vi "on_axis_coupling.vi"(11 "Sense coupling":T1 format="%#_3p") -> (3 "Sense amplitudes":T1 format="%#_3p")   [LabVIEW 2026]
uses:
  coupling_matrix.ctl
panel:
  # "Take a current sense coupling matrix and turn it into one suitable for normalization.   The idea is that only the on-axis source amplitudes are relevant to compensation.  All input channels get the same compensation. So what we are doing is filling each column with the diagonal element."
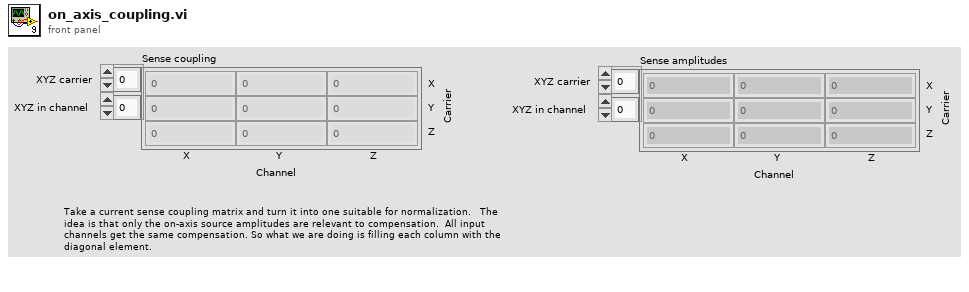
[diagram p1: front panel]
types:
  T1 = typedef "coupling_matrix.ctl" = cdb[][]
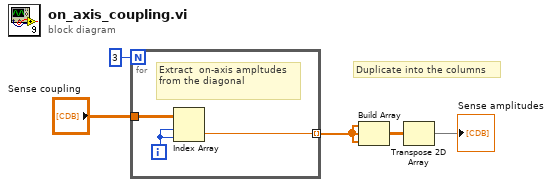
[diagram p0: block diagram]
diagram:
  # "Duplicate into the columns"
  n1 = for {
    N: 3 -> [_]
    tunnel: "Sense coupling" -> [w8]
    tunnel: [w6] -> w3 mode=indexing
    i -> [w7]
    # "Extract  on-axis ampltudes from the diagonal"
    n2 = Index Array(array=w8, index (row)=w7, index (col)=w7) -> (element=w6:cdb)
  }
  n3 = Build Array(w3, w3, w3) -> (w2:cdb[][])
  n4 = Transpose 2D Array(2D array=w2) -> (transposed array=→"Sense amplitudes":cdb[][])
